vi "Launch Step Configuration.vi"(8 "error in (no error)":errorcluster, 11 "Measurement UI in":refnum<class "Measurement UI.lvclass">) -> (0 "error out":errorcluster, 3 "Measurement UI out":refnum<class "Measurement UI.lvclass">)   [LabVIEW 2017, in "Measurement UI.lvlib" / "Measurement UI.lvclass"]
uses:
  Measurement UI.lvclass
  C:/Program Files (x86)/National Instruments/LabVIEW 2017/vi.lib/ActorFramework/Actor/Actor.lvclass
  Measurement UI.lvclass/Measurement UI.ctl
  <vilib>/ActorFramework/Actor/Actor.lvclass/Actor.ctl
  Controller Messages/Launch Step Configuration Msg/Launch Step Configuration Msg.lvclass/Launch Step Configuration Msg.ctl
  <vilib>/ActorFramework/Message Enqueuer/Message Enqueuer.lvclass/Message Enqueuer.ctl
  Accessors/Read Measurement.vi
  <vilib>/ActorFramework/Message Enqueuer/Enqueue.vi
  Controller Messages/Launch Step Configuration Msg/Launch Step Configuration Msg.lvclass
  C:/Program Files (x86)/National Instruments/LabVIEW 2017/vi.lib/ActorFramework/Message/Message.lvclass
  <vilib>/ActorFramework/Message Priority Queue/Priority Enqueue.vi
  <vilib>/ActorFramework/Actor/Actor.lvclass
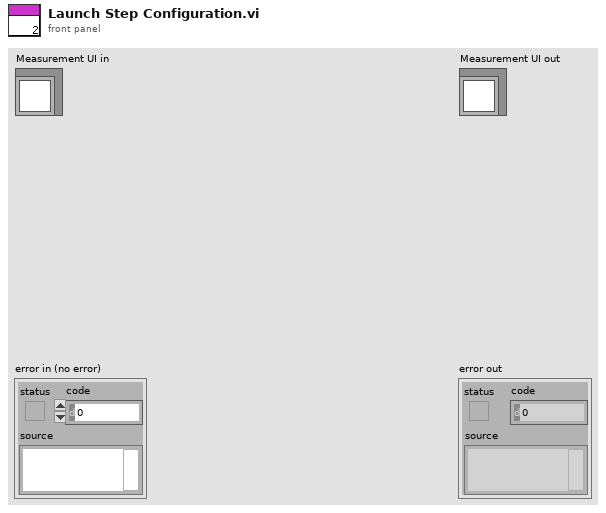
[diagram p1: front panel]
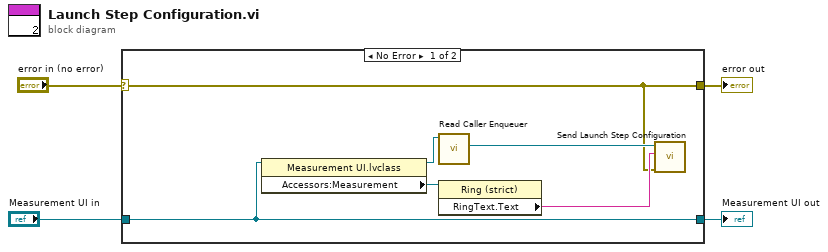
[diagram p0: block diagram]
diagram:
  n1 = case shown="No Error" "error in (no error)" {
    selector: "error in (no error)" -> [w5 w12]
    tunnel: [w5 w12] -> w3
    tunnel: [w8 w11] -> w1
    tunnel: "Measurement UI in" -> [w8 w11]
    frame No Error {
      n2 = property class="Measurement UI.lvclass"(reference=w8) -> (reference out=w10:refnum<class "Measurement UI.lvclass">, "Accessors:Measurement"=w9:refnum<vi>)  [unwired: 1 in, 1 out]
      n3 = call <vilib>:"Read Caller Enqueuer.vi"("Actor"=w10) -> ("Caller Enqueuer"=w7:refnum<class "Message Enqueuer.lvclass">)  [unwired: 10 in]
      n4 = property class="Ring (strict)"(reference=w9) -> ("RingText.Text"=w6:string)  [unwired: 1 in, 2 out]
      n5 = call "Send Launch Step Configuration.vi"("error in (no error)"=w5, "Step Name"=w6, "Message Enqueuer"=w7) -> ()  [unwired: 7 in, 2 out]
    }
    frame Error {
    }
  }
  "error out" <- w3
  "Measurement UI out" <- w1
